vi "Aiming.vi"(6 "PID Cluster":T2={"L1 to L4 PID Cluster"={"L1 PID Gains"={"Kp"=0.005, "Kd"=0.5, "Ki"=0.0005}, "L2 PID Gains"={"Kp"=0.01, "Kd"=1.0, "Ki"=0.005}, "L3 PID Gains"={"Kp"=0.05, "Kd"=1.0, "Ki"=0.0005}, "L4 PID Gains"={"Kp"=0.1, "Kd"=0.1, "Ki"=0.0005}}, "Stage PID Cluster"={"Stage Z PID"={"Kp"=0.0005, "Kd"=0.001, "Ki"=0.0}, "Stage Y PID"={"Kp"=0.0003, "Kd"=0.01, "Ki"=0.0}, "Stage X PID"={"Kp"=0.0003, "Kd"=0.01, "Ki"=0.0}}, "OCT Z PID Gains"={"Kp"=0.0003, "Kd"=0.0001, "Ki"=0.01}}, 7 "Offset Home 2 RCM":dbl[](array[numeric])=[0.0, 0.0, 0.0, 0.0], 8 "error in":errorcluster, 9 "Aiming Pt":dbl[](array[numeric])=[0.0, 0.0, 0.0, 0.0], 10 "Prev Posit Cluster":T3={"Prev L1 to L4 Posit"=[0.0, 0.0, 0.0, 0.0], "Prev Stage Posit"=[6.0, 6.0, 6.0], "Prev OCT Z Posit"=0.0}, 11 "FPGA VI Reference In":refnum<k20>) -> (0 "error out":errorcluster, 2 "Last Posit Cluster":T1={"Last L1 to L4 Posit"=[0.0, 0.0, 0.0, 0.0], "Last Stage Posit"=[6.0, 6.0, 6.0], "Last OCT Z Posit"=0.0}, 3 "FPGA VI Reference Out":refnum<k20>)   [LabVIEW 2016]
uses:
  <vilib>/Platform/TimedLoop/XDataNode/timing_clust.ctl
  <vilib>/Platform/TimedLoop/XDataNode/nitl_modes.ctl
  <vilib>/Platform/TimedLoop/XDataNode/wakeup.ctl
  Global Variables.vi
  <vilib>/platform/TimedLoop/XDataNode/XDataNode.xnode
  <vilib>/Platform/TimedLoop/XDataNode/XDNodeRunTimeDep.lvlib
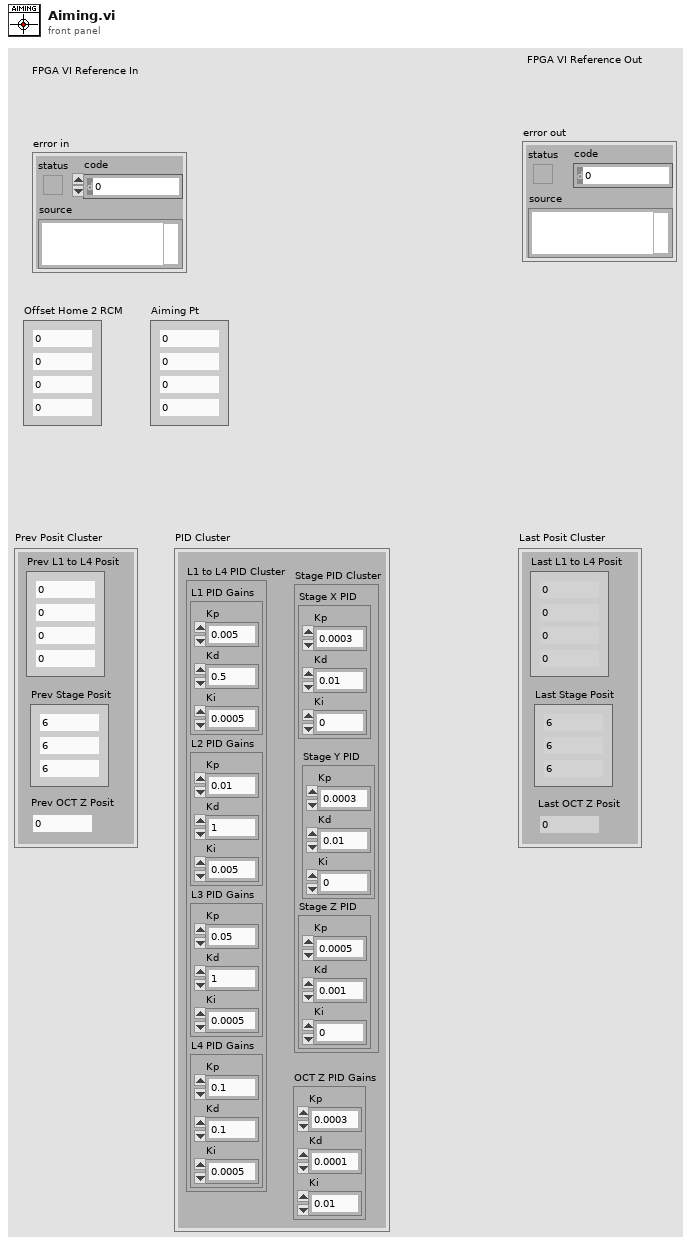
[diagram p1: front panel]
types:
  T1 = cluster{"Last L1 to L4 Posit":dbl[], "Last Stage Posit":dbl[], "Last OCT Z Posit":dbl}
  T2 = cluster{"L1 to L4 PID Cluster":cluster{"L1 PID Gains":cluster{"Kp":dbl, "Kd":dbl, "Ki":dbl}, "L2 PID Gains":cluster{"Kp":dbl, "Kd":dbl, "Ki":dbl}, "L3 PID Gains":cluster{"Kp":dbl, "Kd":dbl, "Ki":dbl}, "L4 PID Gains":cluster{"Kp":dbl, "Kd":dbl, "Ki":dbl}}, "Stage PID Cluster":cluster{"Stage Z PID":cluster{"Kp":dbl, "Kd":dbl, "Ki":dbl}, "Stage Y PID":cluster{"Kp":dbl, "Kd":dbl, "Ki":dbl}, "Stage X PID":cluster{"Kp":dbl, "Kd":dbl, "Ki":dbl}}, "OCT Z PID Gains":cluster{"Kp":dbl, "Kd":dbl, "Ki":dbl}}
  T3 = cluster{"Prev L1 to L4 Posit":dbl[], "Prev Stage Posit":dbl[], "Prev OCT Z Posit":dbl}
  T4 = typedef "XDNodeRunTimeDep.lvlib/timing_clust.ctl" = cluster{"Expected End [f-1]":u64, "Actual End [f-1]":u64, "Finished Late? [f-1]":bool, "Expected End [i-1]":u64, "Actual End [i-1]":u64, "Finished Late? [i-1]":bool, "Expected Start [i]":u64, "Actual Start [i]":u64, "Expected Start [f]":u64, "Actual Start [f]":u64, "Source Name":string, "Structure Name":string, "Period":i64, "Deadline":i64, "Offset":i64, "Start":i64, "Priority":i32, "Timeout":i32, "Mode":T5, "Wakeup Reason":T6, "Error":errorcluster, "Source Type":string, "Secondary Source Type":string, "Global End Time":u64, "Global Start Time":u64, "Frame Duration":u64, "Iteration Duration":u64, "Assigned CPU":i32, "I/O Scan Engine Mode":u32}
  T5 = typedef "XDNodeRunTimeDep.lvlib/nitl_modes.ctl" = enum32{"No Change", "Process missed periods, maintain original phase", "Discard missed periods, maintain original phase", "Process missed periods, ignore original phase", "Discard missed periods, ignore original phase"}
  T6 = typedef "XDNodeRunTimeDep.lvlib/wakeup.ctl" = enum32{"Normal", "Aborted", "Asynchronous wakeup", "Timing source error", "Timed loop error", "Timeout"}
  T7 = cluster{"Stage Z PID":cluster{"Kp":dbl, "Kd":dbl, "Ki":dbl}, "Stage Y PID":cluster{"Kp":dbl, "Kd":dbl, "Ki":dbl}, "Stage X PID":cluster{"Kp":dbl, "Kd":dbl, "Ki":dbl}}
  T8 = cluster{"L1 PID Gains":cluster{"Kp":dbl, "Kd":dbl, "Ki":dbl}, "L2 PID Gains":cluster{"Kp":dbl, "Kd":dbl, "Ki":dbl}, "L3 PID Gains":cluster{"Kp":dbl, "Kd":dbl, "Ki":dbl}, "L4 PID Gains":cluster{"Kp":dbl, "Kd":dbl, "Ki":dbl}}
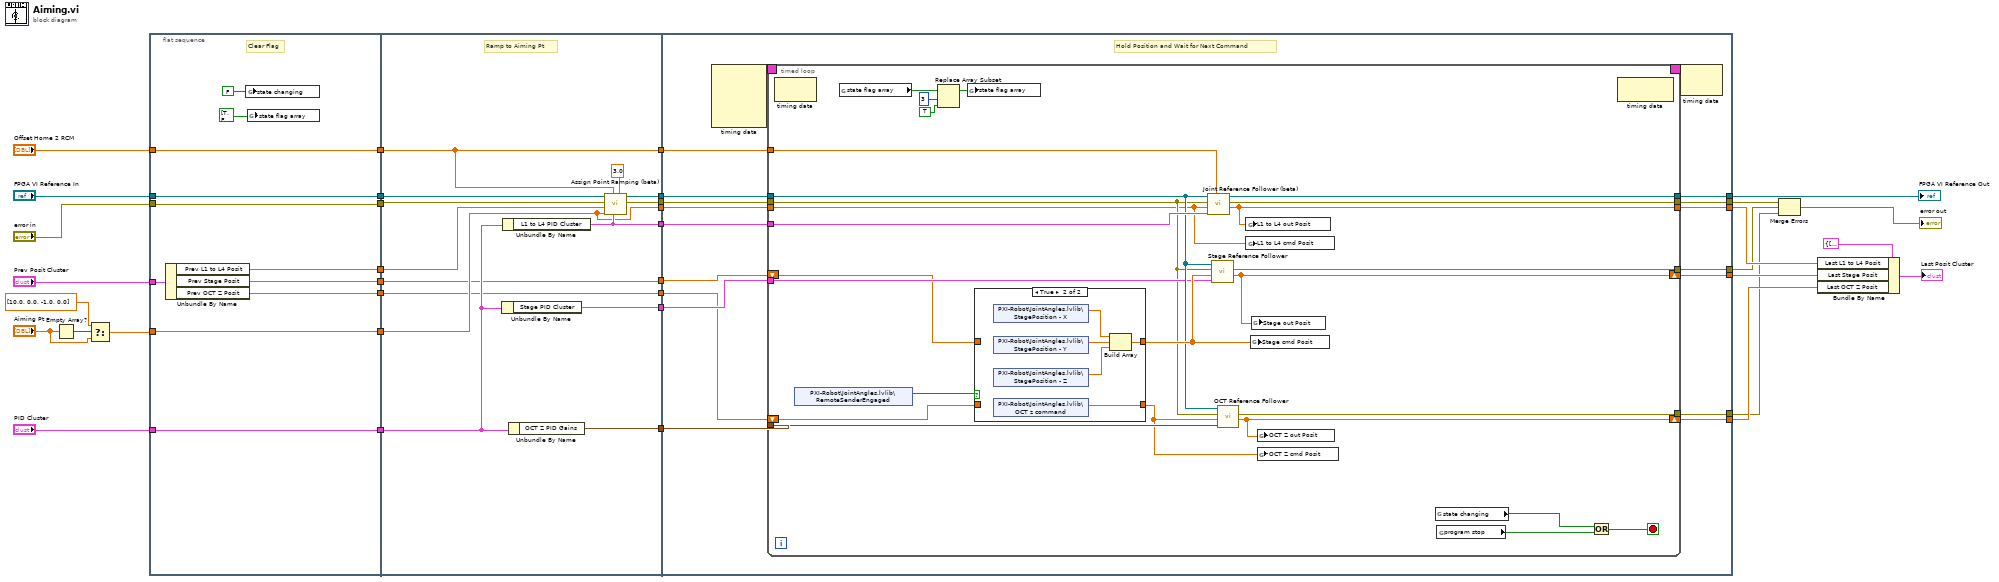
[diagram p0: block diagram]
diagram:
  n1 = Empty Array?(array="Aiming Pt") -> (empty?=w28:bool)
  n2 = Select(t=dbl[] [10.0, 0.0, -1.0, 0.0] ("First Trk Pt 2"), s=w28, f="Aiming Pt") -> (s? t:f=w25:dbl[])
  n3 = flat-sequence {
    tunnel: [w45] -> w36
    tunnel: "FPGA VI Reference In" -> [w45]
    tunnel: "error in" -> [w44]
    tunnel: [w44] -> w35
    tunnel: [w37] -> w34
    tunnel: "PID Cluster" -> [w42]
    tunnel: "Offset Home 2 RCM" -> [w43]
    tunnel: [w43] -> w32
    tunnel: [w38] -> w30
    tunnel: w25 -> [w38]
    tunnel: [w42] -> w18
    tunnel: "Prev Posit Cluster" -> [w41]
    tunnel: [w40] -> w4
    tunnel: [w39] -> w1
    tunnel: w36 -> [w61]
    tunnel: w35 -> [w60]
    tunnel: w34 -> [w58]
    tunnel: w32 -> [w55]
    tunnel: w30 -> [w50]
    tunnel: [w57] -> w29
    tunnel: [w50] -> w24
    tunnel: [w56] -> w23
    tunnel: [w55] -> w22
    tunnel: [w54] -> w21
    tunnel: w18 -> [w52]
    tunnel: [w53] -> w17
    tunnel: [w51] -> w16
    tunnel: w4 -> [w49]
    tunnel: [w49] -> w3
    tunnel: [w48] -> w2
    tunnel: w1 -> [w48]
    tunnel: [w73] -> w12
    tunnel: [w72] -> w7
    tunnel: w29 -> [w76]
    tunnel: w24 -> [w75]
    tunnel: w23 -> [w77]
    tunnel: w22 -> [w64]
    tunnel: w21 -> [w74]
    tunnel: [w71] -> w19
    tunnel: [w70] -> w20
    tunnel: w17 -> [w69]
    tunnel: w16 -> [w68]
    tunnel: [w67] -> w13
    tunnel: [w66] -> w6
    tunnel: [w65] -> w5
    tunnel: w3 -> [w63]
    tunnel: w2 -> [w62]
    frame #0 {
      # "Clear Flag"
      n4 = Unbundle By Name(w41) -> ("Prev L1 to L4 Posit"=w37:dbl[], "Prev Stage Posit"=w40:dbl[], "Prev OCT Z Posit"=w39:dbl)
      n5 = global write "Global Variables.vi" "state changing"(FALSE ("state changing")) -> ()
      n6 = global write "Global Variables.vi" "state flag array"(bool[] [TRUE, FALSE, FALSE, FALSE, FALSE, FALSE, FALSE, FALSE, FALSE] ("state flag array")) -> ()
    }
    frame #1 {
      # "Ramp to Aiming Pt"
      n7 = Unbundle By Name(w52) -> ("Stage PID Cluster"=w53:T7)
      n8 = Unbundle By Name(w52) -> ("L1 to L4 PID Cluster"=w54:T8)
      n9 = Unbundle By Name(w52) -> ("OCT Z PID Gains"=w51:cluster{"Kp":dbl, "Kd":dbl, "Ki":dbl})
      n10 = call "Assign Point Ramping (beta).vi"("Ramp Time [sec]"=3.0, "L1 to L4 PID Cluster"=w54, "Offset Home2RCM"=w55, "Destination Posit Array [mm]"=w50, "Previous Posit Array"=w58, "error in"=w60, "FPGA VI Reference In"=w61) -> ("error out"=w57:errorcluster, "FPGA VI Reference Out"=w56:refnum<k20>)  [unwired: 2 in, 1 out]
    }
    frame #2 {
      # "Hold Position and Wait for Next Command"
      n11 = node-c288() -> (w79:T4)  [unwired: 4 in]
      n12 = timed-loop {
        timing: w79 -> [_]
        timing-out: [_] -> w78
        tunnel: w77 -> [w94]
        tunnel: w76 -> [w86]
        tunnel: w64 -> [w100]
        tunnel: w75 -> [w80]
        tunnel: w74 -> [w99]
        tunnel: [w98] -> w73
        tunnel: [w97] -> w72
        tunnel: [w92] -> w71
        tunnel: w69 -> [w91]
        tunnel: w68 -> [w90]
        tunnel: [w85] -> w66
        tunnel: [w84] -> w65
        shift-right: [w95] -> w70
        shift-left: w63 -> [w82]
        shift-right: [w89] -> w67
        shift-left: w62 -> [w81]
        stop <- w87 stop-if-true
        n13 = node-c288() -> ()  [unwired: 1 in, 1 out]
        n14 = shared-variable "PXI-Robot\\JointAngles.lvlib\\RemoteSenderEngaged"() -> (w83:bool)  [unwired: 1 in, 1 out]
        n15 = global read "Global Variables.vi" "state flag array"() -> (w104:bool[])
        n16 = Replace Array Subset(array=w104, new element=TRUE ("new element/subarray"), index=3) -> (w103:bool[])
        n17 = global write "Global Variables.vi" "state flag array"(w103) -> ()
        n18 = case shown="True" w83 {
          tunnel: [w107 w109] -> w96
          tunnel: [w106 w108] -> w88
          tunnel: w82 -> [w107 _]
          tunnel: w81 -> [w106 _]
          frame False {
            # "Hold Position if not Engaged"
          }
          frame True {
            n19 = shared-variable "PXI-Robot\\JointAngles.lvlib\\StagePosition - X"() -> (w112:dbl)  [unwired: 1 in, 1 out]
            n20 = shared-variable "PXI-Robot\\JointAngles.lvlib\\StagePosition - Y"() -> (w111:dbl)  [unwired: 1 in, 1 out]
            n21 = shared-variable "PXI-Robot\\JointAngles.lvlib\\StagePosition - Z"() -> (w110:dbl)  [unwired: 1 in, 1 out]
            n22 = shared-variable "PXI-Robot\\JointAngles.lvlib\\OCT z command"() -> (w108:dbl)  [unwired: 1 in, 1 out]
            n23 = Build Array(w112, w111, w110) -> (w109:dbl[])
          }
        }
        n24 = call "Joint Reference Follower (beta).vi"("Offset Home2RCM [deg/mm]"=w100, "PID Ctrl Cluster"=w99, "Ref Array [deg/mm]"=w80, "error in"=w86, "FPGA VI Reference In"=w94) -> ("Output Posit Array [deg/mm]"=w92:dbl[], "error out"=w97:errorcluster, "FPGA VI Reference Out"=w98:refnum<k20>)  [unwired: 4 in]
        n25 = call "Stage Reference Follower.vi"("Stage PID Cluster"=w91, "Stage cmd Posit [mm]"=w96, "error in"=w86, "FPGA VI Reference In"=w94) -> ("Stage out Posit [mm]"=w95:dbl[], "error out"=w85:errorcluster)  [unwired: 5 in, 1 out]
        n26 = call "OCT Reference Follower.vi"("OCT Z PID Gains"=w90, "OCT  Z cmd Posit [mm]"=w88, "error in"=w86, "FPGA VI Reference In"=w94) -> ("OCT  Z out Posit [mm]"=w89:dbl, "error out"=w84:errorcluster)  [unwired: 5 in, 1 out]
        n27 = global write "Global Variables.vi" "L1 to L4 out Posit"(w92) -> ()
        n28 = global write "Global Variables.vi" "L1 to L4 cmd Posit"(w80) -> ()
        n29 = global write "Global Variables.vi" "Stage cmd Posit"(w96) -> ()
        n30 = global write "Global Variables.vi" "Stage out Posit"(w95) -> ()
        n31 = global write "Global Variables.vi" "OCT Z out Posit"(w89) -> ()
        n32 = global write "Global Variables.vi" "OCT Z cmd Posit"(w88) -> ()
        n33 = global read "Global Variables.vi" "state changing"() -> (w105:bool)
        n34 = global read "Global Variables.vi" "program stop"() -> (w93:bool)
        n35 = Or(x=w105, y=w93) -> (x .or. y?=w87:bool)
        n36 = node-c288() -> ()  [unwired: 1 in, 1 out]
      }
      n37 = node-c288(w78) -> ()  [unwired: 1 out]
    }
  }
  n38 = Merge Errors(w7, w6, w5) -> (→"error out":errorcluster)
  n39 = Bundle By Name(cluster=T1 {"Last L1 to L4 Posit"=[0.0, 0.0, 0.0, 0.0], "Last Stage Posit"=[6.0, 6.0, 6.0], "Last OCT Z Posit"=0.0} ("Last Posit Cluster 2"), "Last L1 to L4 Posit"=w19, "Last Stage Posit"=w20, "Last OCT Z Posit"=w13) -> (→"Last Posit Cluster":T1)
  "FPGA VI Reference Out" <- w12
